vi "Encoder Driver.vi"(11 "UI elements cluster":T1) -> (0 "Error out (no error)":errorcluster)   [LabVIEW 2017]
uses:
  Typedefs/Speed logging states enum.ctl
  Typedefs/UI ctrl refs cluster.ctl
  Typedefs/Laser control knob.ctl
  Typedefs/Frame Size.ctl
  Typedefs/Plane Mode.ctl
  Typedefs/PMT control knob.ctl
  User Interface/Misc/Experiment Type.ctl
  User Interface/Misc/Biology Information.ctl
  Typedefs/HW config states enum.ctl
  Typedefs/Speed window notifier data.ctl
  Typedefs/Notifier Function.ctl
  Typedefs/Speed acq notifier data.ctl
  Global Variables/General Globals.vi
  Global Variables/gl_UI Ctrl Refs.vi
  <vilib>/Utility/tcp.llb/UDP Multicast Read-Write Open.vi
panel:
  out "# elements in queue":i32
  out "PC's IP":string
  out "Loop time (ms)":u32
  out "Loop duration uS":i32
  out "timestamp uS":i32
  out "File path & name":path
  out "State":T2
  out "Closed":bool
  in  "Stop":bool
  in  "Start":bool
  out "Logging interval":u32
  out "Interval of returned values":u32
  in  "Sim":bool
  in  "Stop Button":bool
  out "RPM":dbl(knob) scale=-200.0..200.0
  in  "Path":path=path "C:/Microscope data/April 2014/16 April 2014/Images_16_04_2014"
  out "Chart":dbl(graph)
  out "Angle (Deg)":dbl(knob) scale=0.0..360.0
  # "Simulated Logging Trigger"
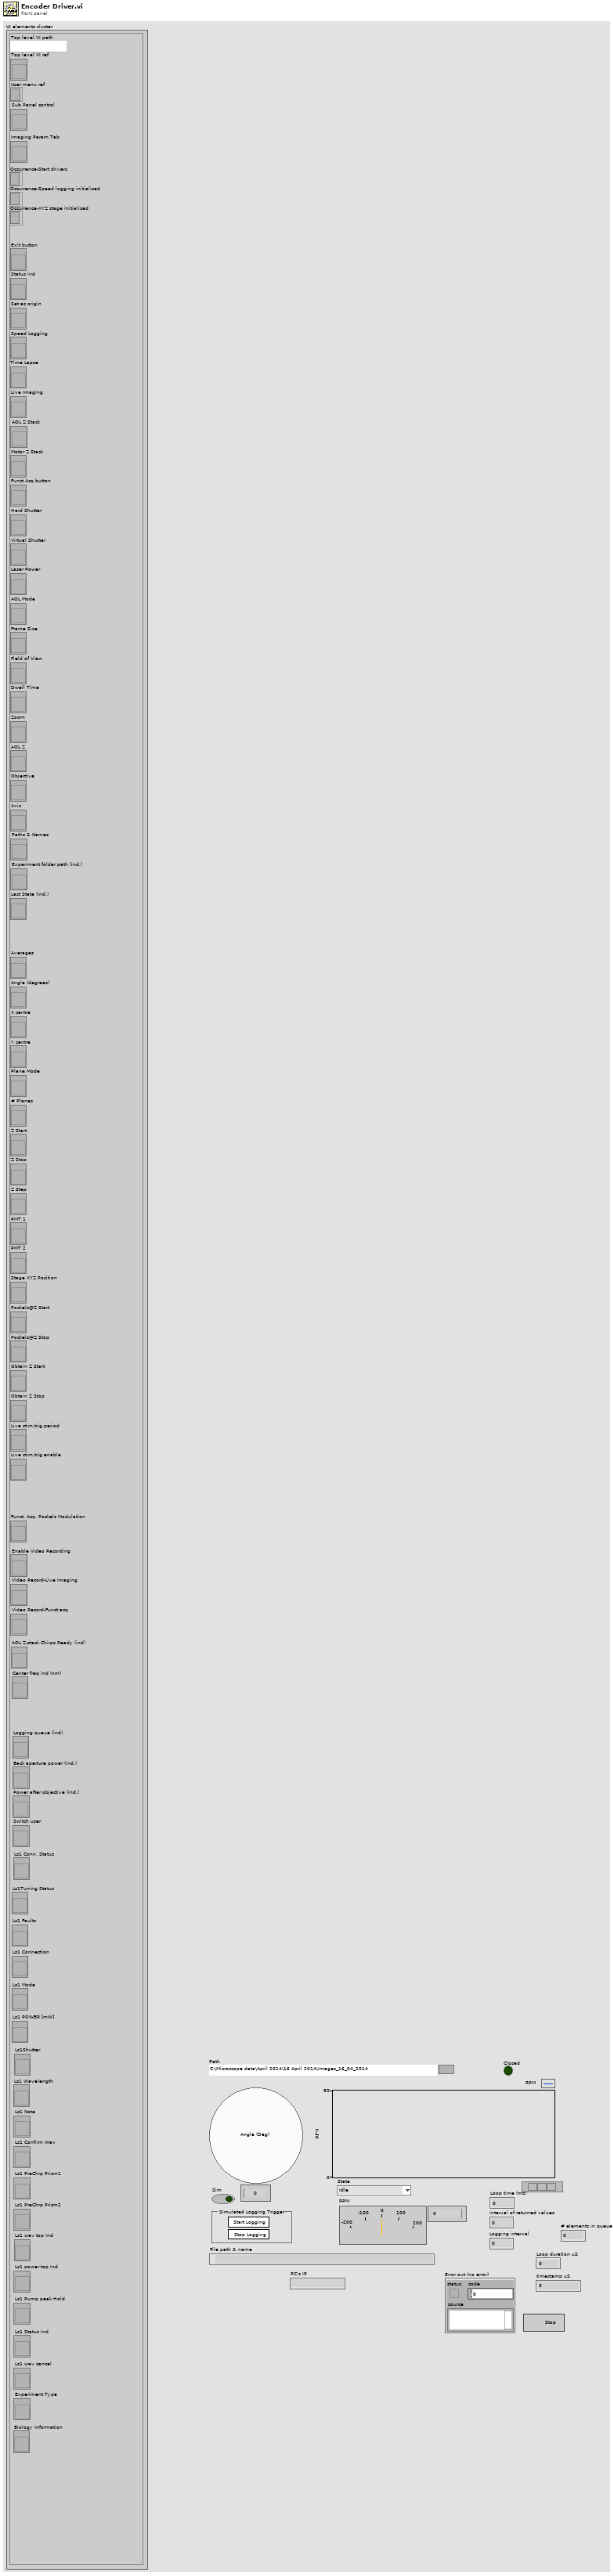
[diagram p1: front panel]
types:
  T1 = typedef "UI ctrl refs cluster.ctl" = cluster{"Top level VI path":path, "Top level VI ref":refnum<vi>, "User menu ref":refnum<k9>, "Sub Panel control":refnum<vi>, "Imaging Param Tab":refnum<vi>, "Occurrence-Start drivers":refnum<k4>, "Occurrence-Speed logging initialised":refnum<k4>, "Occurrence-XYZ stage initialised":refnum<k4>, "Exit button":refnum<vi>, "Status ind":refnum<vi>, "Set as origin":refnum<vi>, "Speed Logging":refnum<vi>, "Time Lapse":refnum<vi>, "Live Imaging":refnum<vi>, "AOL Z Stack":refnum<vi>, "Motor Z Stack":refnum<vi>, "Funct Acq button":refnum<vi>, "Hard Shutter":refnum<vi>, "Virtual Shutter":refnum<vi>, "Laser Power":refnum<vi>, "AOL Mode":refnum<vi>, "Frame Size":refnum<vi>, "Field of View":refnum<vi>, "Dwell Time":refnum<vi>, "Zoom":refnum<vi>, "AOL Z":refnum<vi>, "Objective":refnum<vi>, "Axis":refnum<vi>, "Paths & Names":refnum<vi>, "Experiment folder path (ind.)":refnum<vi>, "Last State (Ind.)":refnum<vi>, "Averages":refnum<vi>, "Angle (degrees)":refnum<vi>, "X centre":refnum<vi>, "Y centre":refnum<vi>, "Plane Mode":refnum<vi>, "# Planes":refnum<vi>, "Z Start":refnum<vi>, "Z Stop":refnum<vi>, "Z Step":refnum<vi>, "PMT 1":refnum<vi>, "PMT 2":refnum<vi>, "Stage XYZ Position":refnum<vi>, "Pockels@Z Start":refnum<vi>, "Pockels@Z Stop":refnum<vi>, "Obtain Z Start":refnum<vi>, "Obtain Z Stop":refnum<vi>, "Live stim.trig.period":refnum<vi>, "Live stim.trig.enable":refnum<vi>, "Funct. Acq. Pockels Modulation":refnum<vi>, "Enable Video Recording":refnum<vi>, "Video Record-Live Imaging":refnum<vi>, "Video Record-Funct acq":refnum<vi>, "AOL Z-stack Chirps Ready (ind)":refnum<vi>, "Center freq ind (nm)":refnum<vi>, "Logging queue (ind)":refnum<vi>, "Back aperture power (ind.)":refnum<vi>, "Power after objective (ind.)":refnum<vi>, "Switch user":refnum<vi>, "Ls1 Conn. Status":refnum<vi>, "Ls1Tuning Status":refnum<vi>, "Ls1 Faults":refnum<vi>, "Ls1 Connection":refnum<vi>, "Ls1 Mode":refnum<vi>, "Ls1 POWER [mW]":refnum<vi>, "Ls1Shutter":refnum<vi>, "Ls1 Wavelength":refnum<vi>, "Ls1 Note":refnum<vi>, "Ls1 Confirm Wav":refnum<vi>, "Ls1 PreChrp Prism1":refnum<vi>, "Ls1 PreChrp Prism2":refnum<vi>, "Ls1 wav top Ind":refnum<vi>, "Ls1 power top Ind":refnum<vi>, "Ls1 Pump peak Hold":refnum<vi>, "Ls1 Status Ind":refnum<vi>, "Ls1 wav cancel":refnum<vi>, "Experiment Type":refnum<vi>, "Biology Information":refnum<vi>}
  T2 = typedef "Speed logging states enum.ctl" = enum16{"Idle", "Open file", "Log", "Close file"}
  T3 = typedef "HW config states enum.ctl" = enum16{"Load from file", "Save to file", "Write all", "Read all", "Write XY stage settings", "Write DAQ FPGA settings", "Write Control FPGA settings", "Write Phys Channels", "Write System Config", "Write HW Config", "Save System Config", "Save HW Config", "Clear", "Compare from file"}
  T4 = typedef "Hardware Configuration settings.ctl" = cluster{"Dev. PC":bool, "Swap XY on stage":bool, "No of AOD":u8, "MC Supported":bool, "Axial MC":bool, "Computer MAC address":string, "Externalise Triggers":bool, "Trigger HW config":T5, "DAQmx Chan":T6, "XY stage available":bool, "XY Stage":T7, "Z stage available":bool, "Z Stage config cluster":T8, "Encoder available":bool, "Encoder":T9, "VidRec available":bool, "Cam VidRec":T10, "Laser Power Control HW config":T11, "Laser 1 available":bool, "Laser 1 config cluster":T12, "Prechirper 1 available":bool, "Prechirper 1 config cluster":T13, "Control system.FPGA available?":bool, "Control Sys. HW config":T14, "DAQ FPGA HW Config":T15}
  T5 = typedef "Triggers HW config.ctl" = cluster{"Available Device List":i32, "Device Address":string}
  T6 = typedef "DAQmx physical channels cluster.ctl" = cluster{"Pockels AO":tag, "Hard shutter AO":tag, "PMT AOs":tag, "Galvo AOs":tag, "Power meter AI":tag}
  T7 = typedef "XY Stage config cluster.ctl" = cluster{"COM port":refnum<visa-resource-name>, "Baudrate":i32, "Type":string}
  T8 = typedef "Z Stage config cluster.ctl" = cluster{"COM port":refnum<visa-resource-name>, "Baudrate":i32, "Type":string}
  T9 = typedef "Encoder config cluster.ctl" = cluster{"IP address":string, "Port":u16, "Wheel radius (cm)":dbl, "Encoder Trigger":tag}
  T10 = typedef "Cam VidRec HW config setup cluster.ctl" = cluster{"DO flag-Video record":tag, "DO flag-Trial start":tag}
  T11 = typedef "Laser Power Control HW config.ctl" = cluster{"Laser Power Control":string, "Laser Power Modulation Control":enum16{"NI", "FPGA"}}
  T12 = typedef "Laser 1 config cluster.ctl" = cluster{"COM port":refnum<visa-resource-name>, "Baud Rate":i32, "Type":string}
  T13 = typedef "PreChirper 1 config cluster.ctl" = cluster{"Type":string, "Baud Rate":i32, "COM port":refnum<visa-resource-name>}
  T14 = typedef "Control Sys HW config cluster.ctl" = cluster{"Control system.FPGA Type":enum16{"Virtex 5", "Virtex 7"}, "Control system.Network adapter name":string, "Control system.MAC address":string, "Control system.Ethernet Port":u32, "Control system.Ethernet Port Opened":bool}
  T15 = typedef "DAQ FPGA HW config cluster.ctl" = cluster{"FGPA Ref":T16, "Target":T17, "input card type":T18}
  T16 = typedef "FPGA Ref.ctl" = refnum<k20>
  T17 = typedef "nirio_resource_hc.ctl" = tag
  T18 = typedef "FPGA input type AC-DC.ctl" = enum16{"AC Card", "DC Card"}
  T19 = typedef "Speed window notifier data.ctl" = cluster{"Angle (Deg)":dbl, "Data value (rpm)":dbl, "Relative time (uS)":i32, "File path":path, "Logging state":T2}
  T20 = typedef "Speed acq notifier data.ctl" = cluster{"Log speed data":bool, "File path":path, "Initial timestamp":timestamp}
  T21 = typedef "Notifier Function.ctl" = enum16{"Send notifier", "Wait on notification", "Release notifier"}
  T22 = enum16{"open", "replace", "create", "open or create", "replace or create", "replace or create with confirmation"}
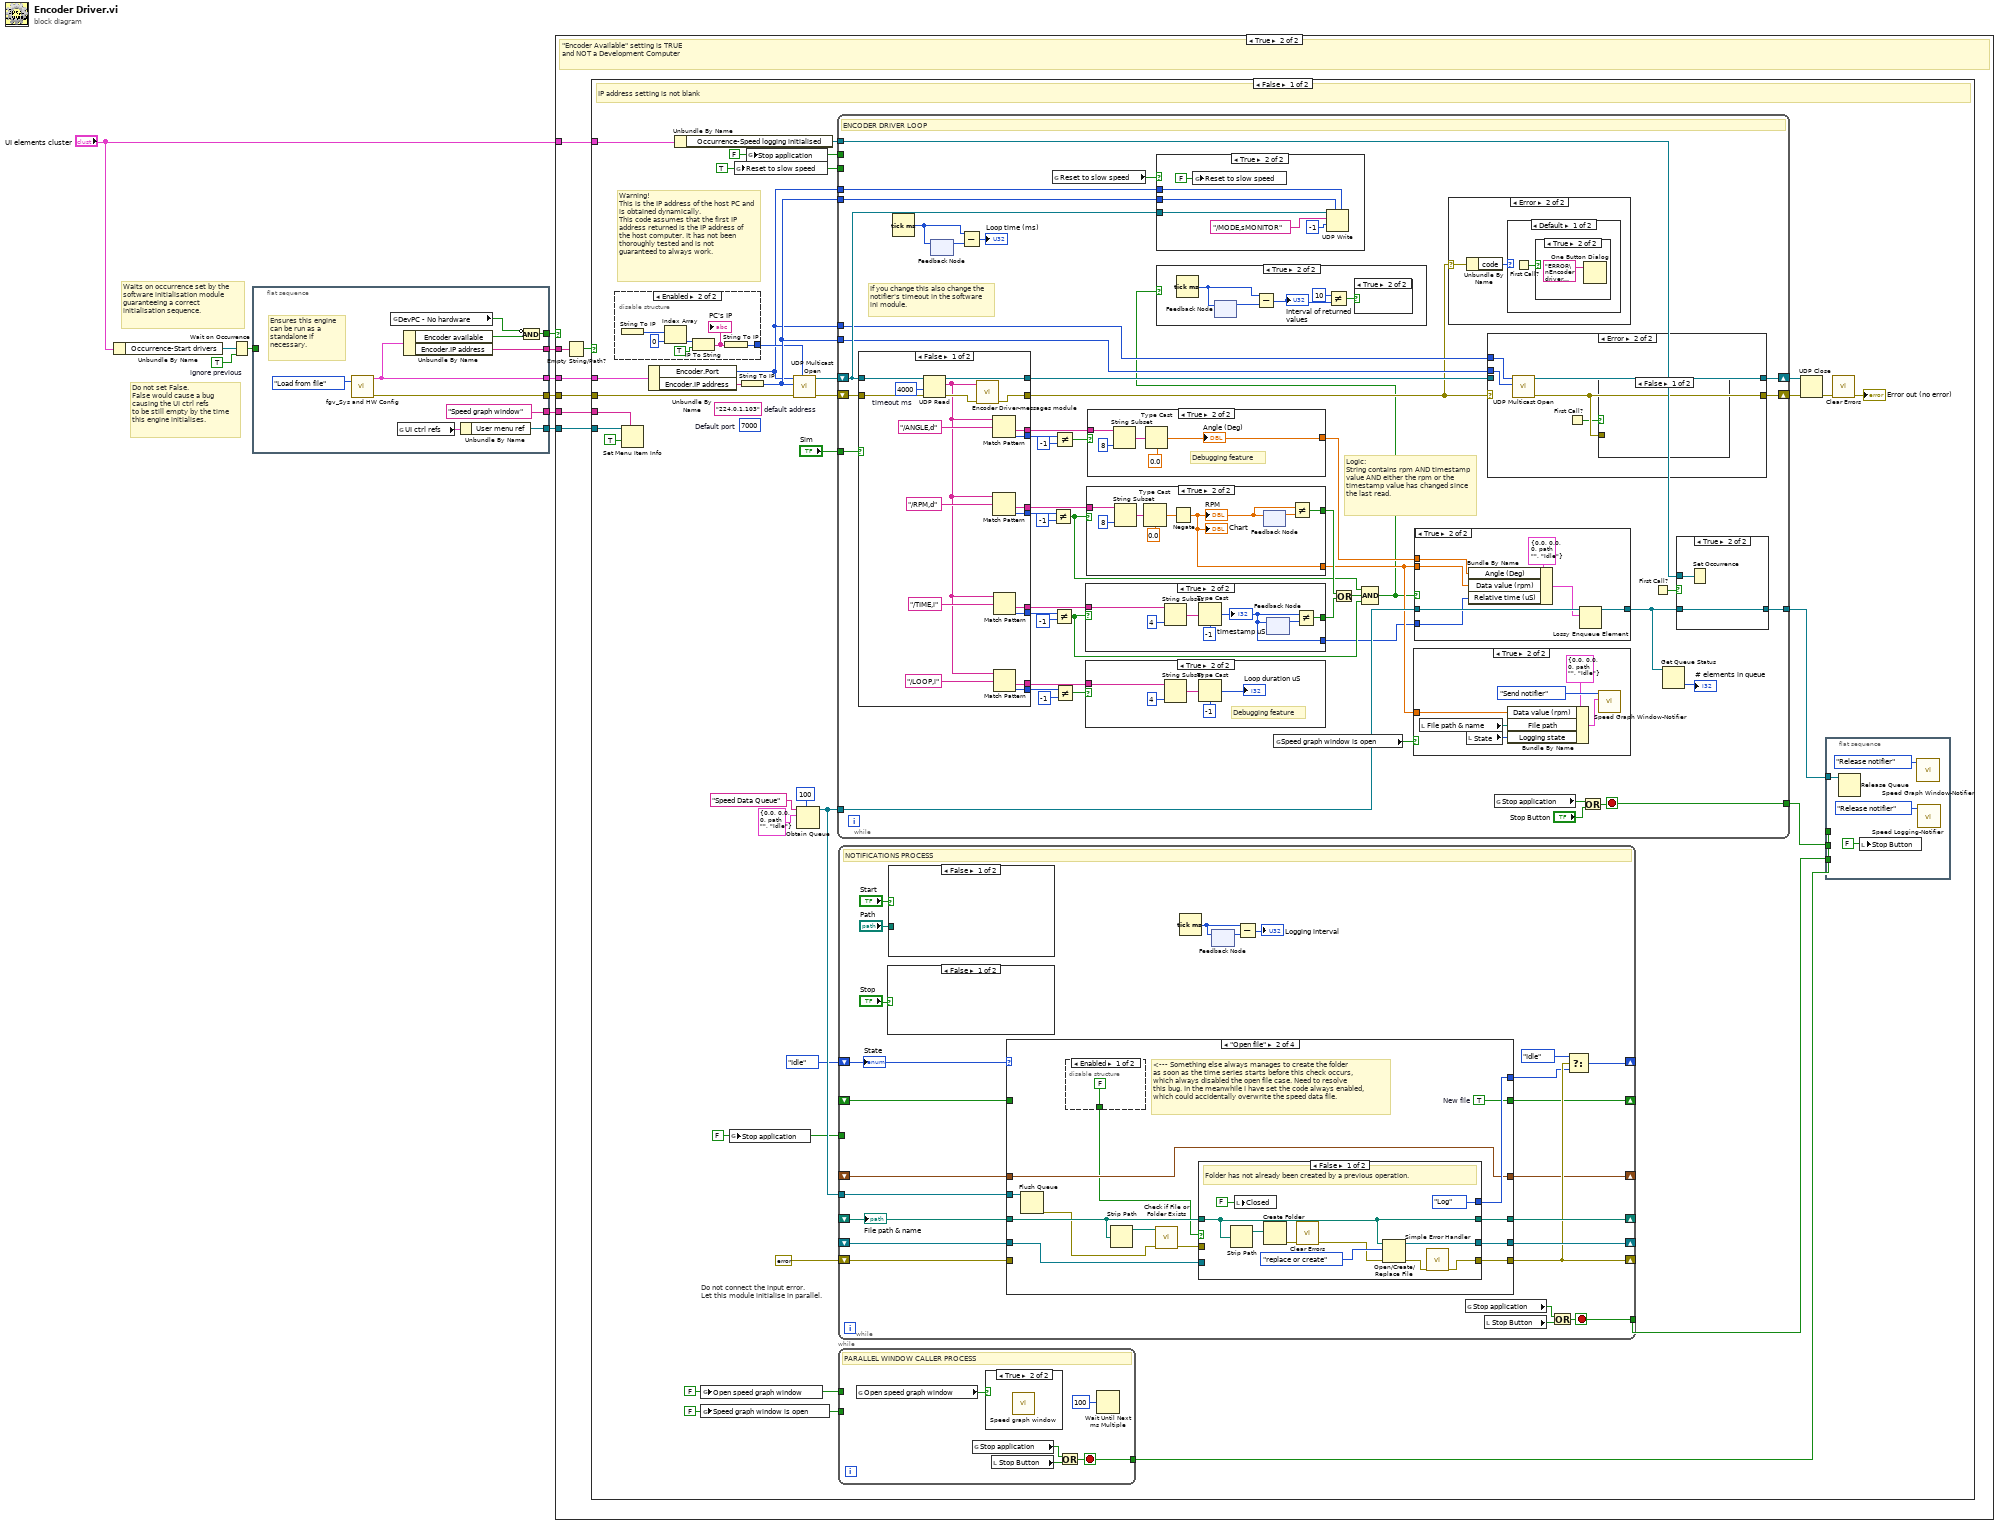
[diagram p0: block diagram]
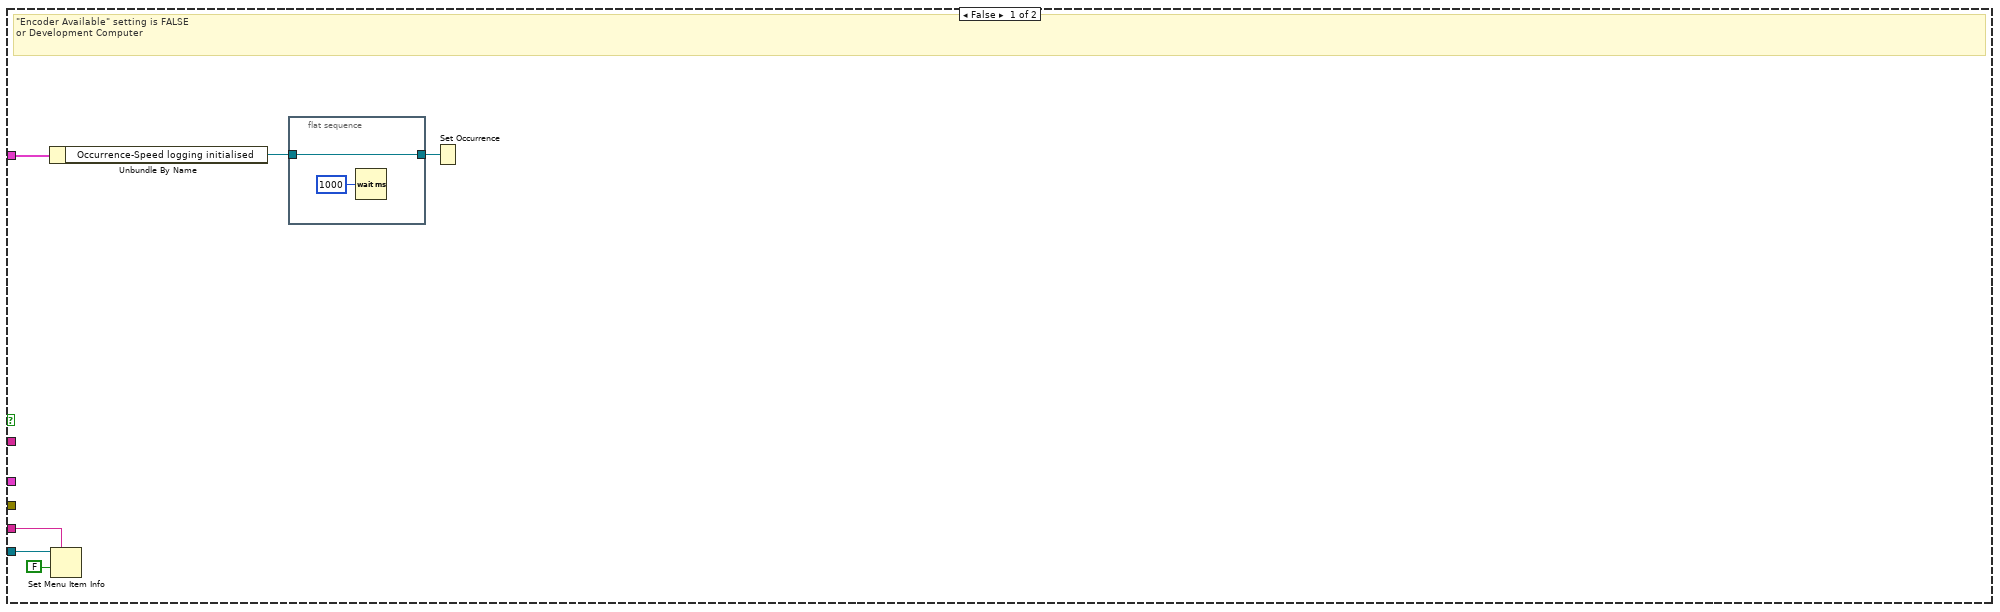
[diagram p2: hidden frame]
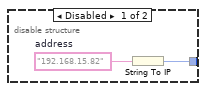
[diagram p3: hidden frame]
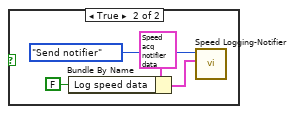
[diagram p5: hidden frame]
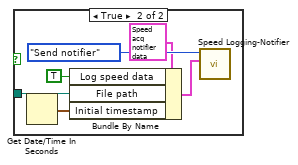
[diagram p6: hidden frame]
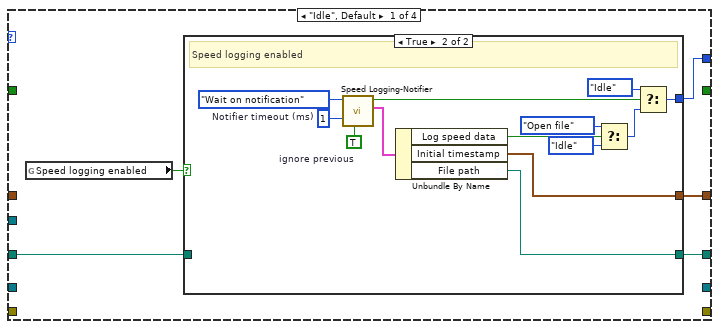
[diagram p7: hidden frame]
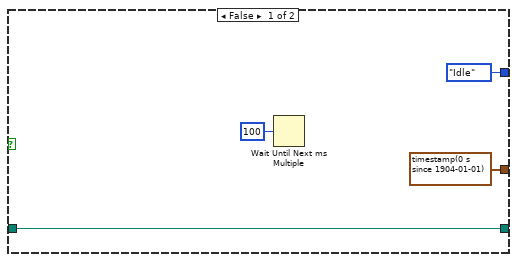
[diagram p8: hidden frame]
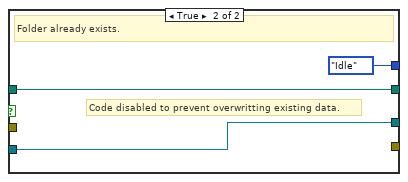
[diagram p10: hidden frame]
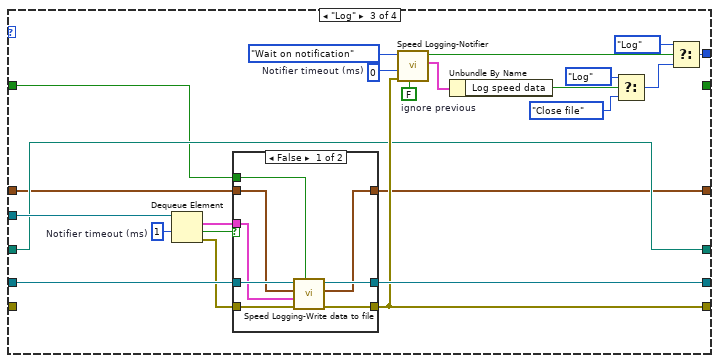
[diagram p11: hidden frame]
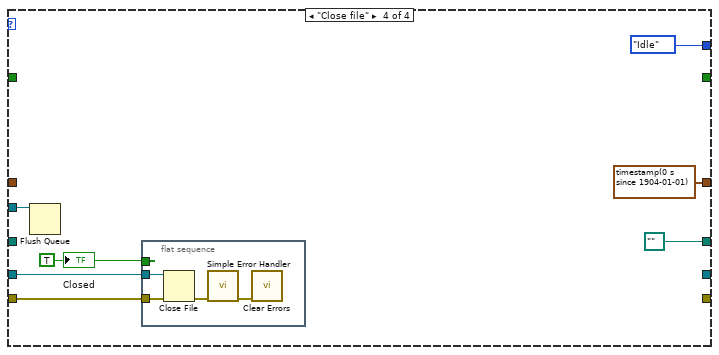
[diagram p13: hidden frame]
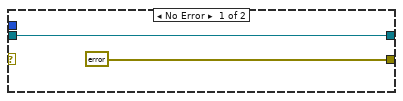
[diagram p14: hidden frame]
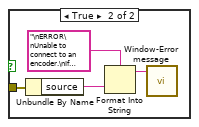
[diagram p15: hidden frame]
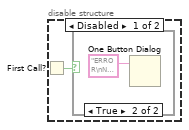
[diagram p20: hidden frame]
diagram:
  w6 = TRUE  # ignore previous
  # "Do not set False.\nFalse would cause a bug\ncausing the UI ctrl refs\nto be still empty by the time\nthis engine initialises."
  # "Waits on occurrence set by the software initialisation module guaranteeing a correct initialisation sequence."
  n1 = Unbundle By Name("UI elements cluster") -> ("Occurrence-Start drivers"=w4:refnum<k4>)
  n2 = Wait on Occurrence(1:w6, 2:w4) -> (0:w5:bool)  [unwired: 1 in]
  n3 = flat-sequence {
    tunnel: [w19] -> w10
    tunnel: [w18] -> w9
    tunnel: [w17] -> w8
    tunnel: [w14] -> w7
    tunnel: w5 -> [_]
    tunnel: [w12] -> w2
    tunnel: ["Speed graph window"] -> w1
    frame #0 {
      # "Ensures this engine can be run as a standalone if necessary."
      n4 = call "fgv_Sys and HW Config.vi"("Function"=HW_config_states_enum."Load from file") -> ("error out"=w19:errorcluster, "Hardware Configuration OUT"=w18:T4)  [unwired: 8 in, 1 out]
      n5 = global read "General Globals.vi" "DevPC - No hardware"() -> (w15:bool)
      n6 = global read "gl_UI Ctrl Refs.vi" "UI ctrl refs"() -> (w13:T1)
      n7 = Unbundle By Name(w18) -> ("Encoder available"=w16:bool, "Encoder.IP address"=w17:string)
      n8 = Unbundle By Name(w13) -> ("User menu ref"=w12:refnum<k9>)
      n9 = Compound Arithmetic op=AND(invert w15, w16) -> (w14:bool)
    }
  }
  n10 = case shown="True" w7 {
    tunnel: "UI elements cluster" -> [w26 w35]
    tunnel: w10 -> [_ w34]
    tunnel: w9 -> [_ w33]
    tunnel: w8 -> [_ w32]
    tunnel: w2 -> [w21 w30]
    tunnel: w1 -> [w22 w29]
    frame False {
      # "\"Encoder Available\" setting is FALSE\nor Development Computer"
      n11 = Unbundle By Name(w26) -> ("Occurrence-Speed logging initialised"=w25:refnum<k4>)
      n12 = Set Menu Item Info(7:w22, 9:FALSE ("enabled"), 11:w21) -> ()  [unwired: 2 in, 4 out]
      n13 = flat-sequence {
        tunnel: w25 -> [w27]
        tunnel: [w27] -> w24
        frame #0 {
          n14 = Wait (ms)(milliseconds to wait=u32 1000) -> ()  [unwired: 1 out]
        }
      }
      n15 = Set Occurrence(w24) -> ()
    }
    frame True {
      # "\"Encoder Available\" setting is TRUE\nand NOT a Development Computer"
      n16 = Empty String/Path?(string/path=w32) -> (empty?=w31:bool)
      n17 = case shown="False" w31 {
        tunnel: w35 -> [w47 _]
        tunnel: w34 -> [w43 _]
        tunnel: w33 -> [w41 _]
        tunnel: w30 -> [w37 w368]
        tunnel: w29 -> [w38 w366]
        frame False {
          w46 = FALSE ("Stop application")
          w58 = TRUE ("Reset to slow speed")
          w53 = FALSE ("Stop application")
          (unwired) u16 7000  # Default port
          (unwired) "224.0.1.103"  # default address
          w51 = FALSE ("Speed graph window is open")
          w52 = FALSE ("Open speed graph window")
          # "Do not connect the input error.\nLet this module initialise in parallel."
          # "Warning!\nThis is the IP address of the host PC and is obtained dynamically.\nThis code assumes that the first IP address returned is the IP address of the host computer. It has not been thoroughly tested and is not guaranteed to always work."
          # "IP address setting is not blank"
          n18 = disable-structure shown="Enabled" {
            disable-tunnel: [w69 w71] -> w50
            frame Disabled {
              w70 = "192.168.15.82"  # address
              n19 = String To IP(1:w70) -> (0:w69:u32)
            }
            frame Enabled {
              n20 = String To IP() -> (0:w72:u32[])  [unwired: 1 in]
              n21 = Index Array(array=w72, index=0) -> (element=w74:u32)
              n22 = IP To String(1:TRUE ("dot notation? (F)"), 2:w74) -> (0:w76:string)
              "PC's IP" <- w76
              n23 = String To IP(1:w76) -> (0:w71:u32)
            }
          }
          n24 = Set Menu Item Info(7:w38, 9:TRUE ("enabled"), 11:w37) -> ()  [unwired: 2 in, 4 out]
          n25 = Unbundle By Name(w41) -> ("Encoder.Port"=w44:u16, "Encoder.IP address"=w45:string)
          n26 = Unbundle By Name(w47) -> ("Occurrence-Speed logging initialised"=w49:refnum<k4>)
          n27 = global write "General Globals.vi" "Open speed graph window"(w52) -> ()
          n28 = global write "General Globals.vi" "Speed graph window is open"(w51) -> ()
          n29 = global write "General Globals.vi" "Stop application"(w53) -> ()
          n30 = global write "General Globals.vi" "Reset to slow speed"(w58) -> ()
          n31 = String To IP(1:w45) -> (0:w57:u32)
          n32 = global write "General Globals.vi" "Stop application"(w46) -> ()
          n33 = call-poly <vilib>:"UDP Multicast Open.vi"("net address"=w50, "error in (no error)"=w43, "multicast addr"=w57, "port"=w44) -> ("error out"=w59:errorcluster, "connection ID"=w62:refnum<k16>)  [unwired: 5 in, 1 out]
          n34 = Obtain Queue(max queue size (-1, unlimited)=100, name (unnamed)="Speed Data Queue", element data type=T19 {"Angle (Deg)"=0.0, "Data value (rpm)"=0.0, "Relative time (uS)"=0, "File path"=path "", "Logging state"=enum."Idle"} ("Speed window data")) -> (queue out=w66:refnum<queue>)  [unwired: 2 in, 2 out]
          n35 = while {
            tunnel: "Sim" -> [w257]
            tunnel: [w252] -> w68
            tunnel: w66 -> [w253]
            tunnel: [w227] -> w65
            tunnel: w57 -> [w250]
            tunnel: w44 -> [w249]
            tunnel: w58 -> [_]
            tunnel: w49 -> [w225]
            tunnel: w57 -> [w223]
            tunnel: w44 -> [w222]
            shift-right: [w221] -> w56
            shift-left: w62 -> [w248]
            shift-right: [w220] -> w55
            shift-left: w59 -> [w228]
            tunnel: w46 -> [_]
            stop <- w252 stop-if-true
            # "If you change this also change the notifier's timeout in the software ini module."
            # "Logic:\nString contains rpm AND timestamp value AND either the rpm or the timestamp value has changed since the last read."
            # "ENCODER DRIVER LOOP"
            n36 = case shown="False" w257 {
              tunnel: w248 -> [w352 w365]
              tunnel: [w350 w362] -> w261
              tunnel: [w348 w365] -> w219
              tunnel: [w347 w360] -> w260
              tunnel: [w345 w360] -> w259
              tunnel: [w344 w362] -> w258
              tunnel: w228 -> [w343 w364]
              tunnel: [w335 w364] -> w218
              tunnel: [w340 w360] -> w246
              tunnel: [w339 w360] -> w244
              tunnel: [w338 w361] -> w243
              tunnel: [w337 w362] -> w242
              frame False {
                w346 = 4000  # timeout ms
                n37 = UDP Read(connection ID=w352, timeout ms (25000)=w346, 8:w343) -> (data out=w334:string, error out=w336:errorcluster, 3:w348:refnum<k16>)  [unwired: 1 in, 2 out]
                n38 = call "Encoder Driver-messages module.vi"("error in (no error)"=w336, "Command/Response string"=w334) -> ("error"=w335:errorcluster)  [unwired: 9 in]
                n39 = Match Pattern(string=w334, regular expression="/ANGLE,d" ("format string")) -> (after substring=w350:string, offset past match=w347:i32)  [unwired: 1 in, 2 out]
                n40 = Match Pattern(string=w334, regular expression="/RPM,d" ("format string")) -> (after substring=w344:string, offset past match=w345:i32)  [unwired: 1 in, 2 out]
                n41 = Match Pattern(string=w334, regular expression="/TIME,i" ("format string")) -> (after substring=w338:string, offset past match=w340:i32)  [unwired: 1 in, 2 out]
                n42 = Match Pattern(string=w334, regular expression="/LOOP,i" ("format string")) -> (after substring=w337:string, offset past match=w339:i32)  [unwired: 1 in, 2 out]
              }
              frame True {
                w360 = 0 ("offset past match")
                n43 = feedback #1() -> (w358:i32)  [unwired: 1 in]
                n44 = Increment(x=w358) -> (x+1=w359:i32)
                n45 = To Long Integer(number=w359) -> (32bit integer=w353:i32)
                n46 = feedback-in #1(w353) -> ()
                n47 = Equal?(x=2147483647 ("32bit integer"), y=w353) -> (x = y?=w356:bool)
                n48 = Random Number (0-1)() -> (number: 0 to 1=w363:dbl)
                n49 = Select(t=0 ("32bit integer"), s=w356, f=w353) -> (s? t:f=w354:i32)
                n50 = Format Into String(w363) -> (resulting string=w362:string)  [unwired: 3 in, 1 out]
                n51 = Format Into String(w354) -> (resulting string=w361:string)  [unwired: 3 in, 1 out]
              }
            }
            n52 = Tick Count (ms)() -> (millisecond timer value=w231:u32)
            n53 = feedback #2() -> (w230:u32)  [unwired: 1 in]
            n54 = feedback-in #2(w231) -> ()
            n55 = Subtract(x=w231, y=w230) -> (x-y=→"Loop time (ms)":u32)
            n56 = Not Equal?(x=w259, y=-1) -> (x != y?=w237:bool)
            n57 = global read "General Globals.vi" "Reset to slow speed"() -> (w232:bool)
            n58 = Not Equal?(x=w246, y=-1) -> (x != y?=w239:bool)
            n59 = Not Equal?(x=w260, y=-1) -> (x != y?=w255:bool)
            n60 = Not Equal?(x=w244, y=-1) -> (x != y?=w241:bool)
            n61 = case shown="True" w239 {
              tunnel: w243 -> [_ w291]
              tunnel: [FALSE w289] -> w240
              tunnel: [_ w288] -> w234
              frame False {
              }
              frame True {
                n62 = String Subset(string=w291, length (rest)=4 ("length (rest)")) -> (substring=w292:string)  [unwired: 1 in]
                n63 = Type Cast(type=-1 ("y"), x=w292) -> (*(type *) &x=w288:i32)
                "timestamp uS" <- w288
                n64 = feedback #3() -> (w290:i32)  [unwired: 1 in]
                n65 = feedback-in #3(w288) -> ()
                n66 = Not Equal?(x=w288, y=w290) -> (x != y?=w289:bool)
              }
            }
            n67 = case shown="True" w241 {
              tunnel: w242 -> [_ w283]
              frame False {
              }
              frame True {
                # "Debugging feature"
                n68 = String Subset(string=w283, length (rest)=4 ("length (rest)")) -> (substring=w284:string)  [unwired: 1 in]
                n69 = Type Cast(type=-1 ("y"), x=w284) -> (*(type *) &x=→"Loop duration uS":i32)
              }
            }
            n70 = case shown="True" w237 {
              tunnel: w258 -> [_ w303]
              tunnel: [FALSE w302] -> w238
              tunnel: [_ w296] -> w235
              frame False {
              }
              frame True {
                n71 = String Subset(string=w303, length (rest)=8 ("length (rest)")) -> (substring=w298:string)  [unwired: 1 in]
                n72 = Type Cast(type=0.0 ("number"), x=w298) -> (*(type *) &x=w297:dbl)
                n73 = Negate(x=w297) -> (-x=w296:dbl)
                "Chart" <- w296
                "RPM" <- w296
                n74 = feedback #4() -> (w300:dbl)  [unwired: 1 in]
                n75 = feedback-in #4(w296) -> ()
                n76 = Not Equal?(x=w296, y=w300) -> (x != y?=w302:bool)
              }
            }
            n77 = case shown="True" w255 {
              tunnel: w261 -> [_ w331]
              tunnel: [_ w329] -> w233
              frame False {
              }
              frame True {
                # "Debugging feature"
                n78 = String Subset(string=w331, length (rest)=8 ("length (rest)")) -> (substring=w330:string)  [unwired: 1 in]
                n79 = Type Cast(type=0.0 ("number"), x=w330) -> (*(type *) &x=w329:dbl)
                "Angle (Deg)" <- w329
              }
            }
            n80 = case shown="True" w232 {
              tunnel: w248 -> [_ w313]
              tunnel: w249 -> [_ w312]
              tunnel: w250 -> [_ w311]
              frame False {
              }
              frame True {
                n81 = global write "General Globals.vi" "Reset to slow speed"(FALSE ("Reset to slow speed")) -> ()
                n82 = UDP Write(address=w311, port or service name=w312, connection ID=w313, data in="/MODE,sMONITOR", 9:-1 ("timeout ms (25000)")) -> ()  [unwired: 1 in, 2 out]
              }
            }
            n83 = global read "General Globals.vi" "Speed graph window is open"() -> (w214:bool)
            n84 = Or(x=w238, y=w240) -> (x .or. y?=w236:bool)
            n85 = Compound Arithmetic op=AND(w237, w236, w239) -> (w215:bool)
            n86 = case shown="True" w215 {
              frame False {
              }
              frame True {
                n87 = Tick Count (ms)() -> (millisecond timer value=w327:u32)
                n88 = feedback #5() -> (w328:u32)  [unwired: 1 in]
                n89 = feedback-in #5(w327) -> ()
                n90 = Subtract(x=w327, y=w328) -> (x-y=w326:u32)
                "Interval of returned values" <- w326
                n91 = Not Equal?(x=u32 10, y=w326) -> (x != y?=w324:bool)
                n92 = case shown="True" w324 {
                  frame False {
                  }
                  frame True {
                  }
                }
              }
            }
            n93 = case shown="True" w214 {
              tunnel: w235 -> [_ w305]
              frame False {
              }
              frame True {
                n94 = local read "File path & name"() -> (w307:path)
                n95 = local read "State"() -> (w304:T2)
                n96 = Bundle By Name(cluster=T19 {"Angle (Deg)"=0.0, "Data value (rpm)"=0.0, "Relative time (uS)"=0, "File path"=path "", "Logging state"=enum."Idle"} ("Speed window data"), "Data value (rpm)"=w305, "File path"=w307, "Logging state"=w304) -> (w306:T19)
                n97 = call "Speed Graph Window-Notifier.vi"("Speed window data"=w306, "Notifier Function"=Notifier_Function."Send notifier") -> ()  [unwired: 7 in, 3 out]
              }
            }
            n98 = case shown="True" w215 {
              tunnel: w253 -> [w316 w323]
              tunnel: [w316 w322] -> w217
              tunnel: w235 -> [_ w319]
              tunnel: w234 -> [_ w318]
              tunnel: w233 -> [_ w317]
              frame False {
              }
              frame True {
                n99 = Bundle By Name(cluster=T19 {"Angle (Deg)"=0.0, "Data value (rpm)"=0.0, "Relative time (uS)"=0, "File path"=path "", "Logging state"=enum."Idle"} ("Speed window data"), "Angle (Deg)"=w317, "Data value (rpm)"=w319, "Relative time (uS)"=w318) -> (w320:T19)
                n100 = Lossy Enqueue Element(queue=w323, element=w320) -> (queue out=w322:refnum<queue>)  [unwired: 1 in, 3 out]
              }
            }
            n101 = case shown="Error" w218 {
              selector: w218 -> [_ w277]
              frame No Error {
              }
              frame Error {
                n102 = Unbundle By Name(w277) -> ("code"=w276:i32)
                n103 = case shown="Default" w276 {
                  frame Default {
                    n104 = First Call?() -> (First Call?: T/F=w278:bool)
                    n105 = case shown="True" w278 {
                      frame False {
                      }
                      frame True {
                        n106 = One Button Dialog(message="ERROR\nEncoder driver comms error.") -> ()  [unwired: 1 in, 1 out]
                      }
                    }
                  }
                  frame 56 {
                    n107 = disable-structure shown="Enabled" {
                      frame Disabled {
                        n108 = First Call?() -> (First Call?: T/F=w280:bool)
                        n109 = case shown="True" w280 {
                          frame False {
                          }
                          frame True {
                            n110 = One Button Dialog(message="ERROR\nNo encoder present.") -> ()  [unwired: 1 in, 1 out]
                          }
                        }
                      }
                      frame Enabled {
                      }
                    }
                  }
                }
              }
            }
            n111 = case shown="Error" w218 {
              tunnel: w223 -> [_ w268]
              tunnel: w222 -> [_ w267]
              tunnel: [w263 w266] -> w221
              tunnel: [errorcluster {"status"=FALSE, "code"=0, "source"=""} ("error out") w265] -> w220
              tunnel: w219 -> [w263 _]
              frame No Error {
              }
              frame Error {
                n112 = call-poly <vilib>:"UDP Multicast Open.vi"("multicast addr"=w268, "port"=w267) -> ("error out"=w265:errorcluster, "connection ID"=w266:refnum<k16>)  [unwired: 7 in, 1 out]
                n113 = First Call?() -> (First Call?: T/F=w264:bool)
                n114 = case shown="False" w264 {
                  tunnel: w265 -> [_ w272]
                  frame False {
                  }
                  frame True {
                    n115 = Unbundle By Name(w272) -> ("source"=w271:string)
                    n116 = Format Into String(format string="\nERROR\nUnable to connect to an encoder.\nIf there is an encoder physically connected to the system carry out the following steps to rectify the issue:\n1. Shut down the software.\n2. Power down the AOL control unit and the encoder driver unit by disconnecting its USB power supply cable.\n3. Power up the encoder driver unit and wait until its LED becomes green.\n4. Start the software.\n5. Power up the AOL control unit and wait for 10 seconds before you use the software for imaging.\n\nERROR SOURCE:\n%s\n\nCheck the firewall!", w271) -> (resulting string=w270:string)  [unwired: 2 in, 1 out]
                    n117 = call "Window-Error message.vi"("Message"=w270) -> ()  [unwired: 10 in, 1 out]
                  }
                }
              }
            }
            n118 = global read "General Globals.vi" "Stop application"() -> (w224:bool)
            n119 = Or(x=w224, y="Stop Button") -> (x .or. y?=w252:bool)
            n120 = First Call?() -> (First Call?: T/F=w226:bool)
            n121 = Get Queue Status(queue=w217) -> (# elements in queue=→"# elements in queue":i32)  [unwired: 2 in, 7 out]
            n122 = case shown="True" w226 {
              tunnel: w217 -> [w273 w275]
              tunnel: [w273 w275] -> w227
              tunnel: w225 -> [_ w274]
              frame False {
              }
              frame True {
                n123 = Set Occurrence(w274) -> ()
              }
            }
          }
          n124 = while {
            tunnel: w52 -> [_]
            tunnel: w51 -> [_]
            tunnel: [w77] -> w40
            stop <- w77 stop-if-true
            # "PARALLEL WINDOW CALLER PROCESS"
            n125 = global read "General Globals.vi" "Open speed graph window"() -> (w78:bool)
            n126 = global read "General Globals.vi" "Stop application"() -> (w80:bool)
            n127 = case shown="True" w78 {
              frame False {
              }
              frame True {
                n128 = call "Speed graph window.vi"() -> ()  [unwired: 12 in]
              }
            }
            n129 = local read "Stop Button"() -> (w81:bool)
            n130 = Or(x=w80, y=w81) -> (x .or. y?=w77:bool)
            n131 = Wait Until Next ms Multiple(millisecond multiple=u32 100 ("millisecond timer value")) -> ()  [unwired: 1 out]
          }
          n132 = while {
            shift-right: [w104] -> _
            shift-left: _ -> [w103]
            shift-right: [w99] -> _
            shift-left: errorcluster {"status"=FALSE, "code"=0, "source"=""} ("error in (no error)") -> [w102]
            shift-right: [w98] -> _
            shift-left: Speed_logging_states_enum."Idle" ("States") -> [w105]
            shift-right: [w101] -> _
            shift-left: _ -> [w100]
            tunnel: [w88] -> w67
            tunnel: w66 -> [w91]
            shift-right: [w84] -> _
            shift-left: _ -> [w85]
            shift-right: [w83] -> _
            shift-left: _ -> [w82]
            tunnel: w53 -> [_]
            stop <- w88 stop-if-true
            # "NOTIFICATIONS PROCESS"
            n133 = case shown="False" "Stop" {
              frame False {
              }
              frame True {
                n134 = Bundle By Name(cluster=T20 {"Log speed data"=TRUE, "File path"=path "", "Initial timestamp"=timestamp(0 s since 1904-01-01)} ("Value to send"), "Log speed data"=FALSE ("Log?")) -> (w106:T20)
                n135 = call "Speed Logging-Notifier.vi"("Value to send"=w106, "Notifier Function"=Notifier_Function."Send notifier") -> ()  [unwired: 7 in, 3 out]
              }
            }
            n136 = case shown="False" "Start" {
              tunnel: "Path" -> [_ w112]
              frame False {
              }
              frame True {
                n137 = Get Date/Time In Seconds() -> (seconds since 1Jan1904=w110:timestamp)
                n138 = Bundle By Name(cluster=T20 {"Log speed data"=TRUE, "File path"=path "", "Initial timestamp"=timestamp(0 s since 1904-01-01)} ("Value to send"), "Log speed data"=TRUE ("Log?"), "File path"=w112, "Initial timestamp"=w110) -> (w111:T20)
                n139 = call "Speed Logging-Notifier.vi"("Value to send"=w111, "Notifier Function"=Notifier_Function."Send notifier") -> ()  [unwired: 7 in, 3 out]
              }
            }
            n140 = case shown="\"Open file\"" w105 {
              tunnel: [_ w150 w187 _] -> w104
              tunnel: w103 -> [_ w138 w186 w204]
              tunnel: [_ w149 w178 _] -> w99
              tunnel: w102 -> [_ _ _ w203]
              tunnel: [w120 w147 w179 Speed_logging_states_enum."Idle" ("States")] -> w97
              tunnel: [w119 w148 w169 path "" ("appended path")] -> w101
              tunnel: w100 -> [w118 w145 w169 _]
              tunnel: w91 -> [_ w140 w177 w199]
              tunnel: w85 -> [_ w143 w166 _]
              tunnel: [w116 w143 w165 timestamp(0 s since 1904-01-01) ("seconds since 1Jan1904")] -> w84
              tunnel: [_ w142 _ _] -> w83
              tunnel: w82 -> [_ _ w167 _]
              frame "Idle", Default {
                n141 = global read "General Globals.vi" "Speed logging enabled"() -> (w117:bool)
                n142 = case shown="True" w117 {
                  tunnel: [Speed_logging_states_enum."Idle" ("f") w137] -> w120
                  tunnel: [w123 w125] -> w119
                  tunnel: w118 -> [w123 _]
                  tunnel: [timestamp(0 s since 1904-01-01) ("seconds since 1Jan1904") w126] -> w116
                  frame False {
                    n143 = Wait Until Next ms Multiple(millisecond multiple=u32 100) -> ()  [unwired: 1 out]
                  }
                  frame True {
                    w127 = 1  # Notifier timeout (ms)
                    w130 = TRUE  # ignore previous
                    # "Speed logging enabled"
                    n144 = call "Speed Logging-Notifier.vi"("ignore previous (F)"=w130, "Timeout waiting in ms (-1)"=w127, "Notifier Function"=Notifier_Function."Wait on notification") -> ("Notification data received"=w129:T20, "Timed out waiting"=w131:bool)  [unwired: 6 in, 1 out]
                    n145 = Unbundle By Name(w129) -> ("Log speed data"=w128:bool, "Initial timestamp"=w126:timestamp, "File path"=w125:path)
                    n146 = Select(t=Speed_logging_states_enum."Open file" ("f"), s=w128, f=Speed_logging_states_enum."Idle") -> (s? t:f=w133:T2)
                    n147 = Select(t=Speed_logging_states_enum."Idle" ("States"), s=w131, f=w133) -> (s? t:f=w137:T2)
                  }
                }
              }
              frame "Open file" {
                w142 = TRUE  # New file
                # "<--- Something else always manages to create the folder\nas soon as the time series starts before this check occurs,\nwhich always disabled the open file case. Need to resolve\nthis bug. In the meanwhile I have set the code always enabled,\nwhich could accidentally overwrite the speed data file."
                n148 = Flush Queue(queue=w140) -> (error out=w139:errorcluster)  [unwired: 1 in, 2 out]
                n149 = disable-structure shown="Enabled" {
                  disable-tunnel: [FALSE _] -> w141
                  frame Enabled {
                  }
                  frame Disabled {
                  }
                }
                n150 = Strip Path(path=w145) -> (stripped path=w144:path)  [unwired: 1 out]
                n151 = call <vilib>:"Check if File or Folder Exists.vi"("error in (no error)"=w139, "path"=w144) -> ("error out"=w146:errorcluster)  [unwired: 7 in, 2 out]
                n152 = case shown="False" w141 {
                  tunnel: [w160 w162] -> w150
                  tunnel: [w158 _] -> w149
                  tunnel: [w153 w164] -> w148
                  tunnel: w145 -> [w153 w164]
                  tunnel: [Speed_logging_states_enum."Log" ("States") Speed_logging_states_enum."Idle" ("States")] -> w147
                  tunnel: w146 -> [_ _]
                  tunnel: w138 -> [_ w162]
                  frame False {
                    # "Folder has not already been created by a previous operation."
                    n153 = Strip Path(path=w153) -> (stripped path=w154:path)  [unwired: 1 out]
                    n154 = local write "Closed"(FALSE ("Closed")) -> ()
                    n155 = Create Folder(path (use dialog)=w154) -> (error out=w157:errorcluster)  [unwired: 2 in, 2 out]
                    n156 = call <vilib>:"Clear Errors.vi"("error in (no error)"=w157) -> ("error out"=w152:errorcluster)  [unwired: 5 in, 1 out]
                    n157 = Open/Create/Replace File(file path (use dialog)=w153, error in=w152, operation (0:open)=T22."replace or create") -> (refnum out=w160:refnum<file>, error out=w159:errorcluster)  [unwired: 3 in, 1 out]
                    n158 = call <vilib>:"Simple Error Handler.vi"("error in (no error)"=w159) -> ("error out"=w158:errorcluster)  [unwired: 4 in, 4 out]
                  }
                  frame True {
                    # "Code disabled to prevent overwritting existing data."
                    # "Folder already exists."
                  }
                }
              }
              frame "Log" {
                w172 = 0  # Notifier timeout (ms)
                w173 = 1  # Notifier timeout (ms)
                w176 = FALSE  # ignore previous
                n159 = Dequeue Element(queue=w177, timeout in ms (-1)=w173) -> (element=w168:T19, timed out?=w171:bool, error out=w170:errorcluster)  [unwired: 1 in, 1 out]
                n160 = case shown="False" w171 {
                  tunnel: [w195 w197] -> w187
                  tunnel: w186 -> [w194 w197]
                  tunnel: [w193 w198] -> w178
                  tunnel: w170 -> [w192 w198]
                  tunnel: w168 -> [w191 _]
                  tunnel: w166 -> [w190 w196]
                  tunnel: w167 -> [w189 _]
                  tunnel: [w188 w196] -> w165
                  frame False {
                    n161 = call "Speed Logging-Write data to file.vi"("New file"=w189, "error in (no error)"=w192, "Speed window data"=w191, "Timestamp at trial start"=w190, "Byte Stream File in"=w194) -> ("error out"=w193:errorcluster, "Timestamp at trial start"=w188:timestamp, "Byte Stream File out"=w195:refnum<file>)  [unwired: 4 in]
                  }
                  frame True {
                  }
                }
                n162 = call "Speed Logging-Notifier.vi"("ignore previous (F)"=w176, "error in"=w178, "Timeout waiting in ms (-1)"=w172, "Notifier Function"=Notifier_Function."Wait on notification") -> ("Notification data received"=w175:T20, "Timed out waiting"=w180:bool)  [unwired: 5 in, 1 out]
                n163 = Unbundle By Name(w175) -> ("Log speed data"=w174:bool)
                n164 = Select(t=Speed_logging_states_enum."Log" ("f"), s=w174, f=Speed_logging_states_enum."Close file" ("States")) -> (s? t:f=w182:T2)
                n165 = Select(t=Speed_logging_states_enum."Log", s=w180, f=w182) -> (s? t:f=w179:T2)
              }
              frame "Close file" {
                w202 = TRUE
                n166 = Flush Queue(queue=w199) -> ()  [unwired: 1 in, 3 out]
                n167 = flat-sequence {
                  tunnel: w204 -> [w209]
                  tunnel: w203 -> [w208]
                  tunnel: w202 -> [_]
                  frame #0 {
                    n168 = Close File(refnum=w209, error in=w208) -> (error out=w207:errorcluster)  [unwired: 1 out]
                    n169 = call <vilib>:"Simple Error Handler.vi"("error in (no error)"=w207) -> ("error out"=w206:errorcluster)  [unwired: 4 in, 4 out]
                    n170 = call <vilib>:"Clear Errors.vi"("error in (no error)"=w206) -> ()  [unwired: 5 in, 2 out]
                  }
                }
                "Closed" <- w202
              }
            }
            n171 = Tick Count (ms)() -> (millisecond timer value=w94:u32)
            n172 = feedback #6() -> (w95:u32)  [unwired: 1 in]
            n173 = feedback-in #6(w94) -> ()
            n174 = Subtract(x=w94, y=w95) -> (x-y=→"Logging interval":u32)
            n175 = global read "General Globals.vi" "Stop application"() -> (w90:bool)
            n176 = local read "Stop Button"() -> (w89:bool)
            n177 = Or(x=w90, y=w89) -> (x .or. y?=w88:bool)
            n178 = Select(t=Speed_logging_states_enum."Idle" ("States"), s=w99, f=w97) -> (s? t:f=w98:T2)
            "State" <- w105
            "File path & name" <- w100
          }
          n179 = UDP Close(connection ID=w56, 8:w55) -> (error out=w60:errorcluster)  [unwired: 1 out]
          n180 = flat-sequence {
            tunnel: w68 -> [_]
            tunnel: w67 -> [_]
            tunnel: w65 -> [w211]
            tunnel: w40 -> [_]
            frame #0 {
              n181 = Release Queue(queue=w211) -> ()  [unwired: 2 in, 3 out]
              n182 = local write "Stop Button"(FALSE ("Stop Button")) -> ()
              n183 = call "Speed Graph Window-Notifier.vi"("Notifier Function"=Notifier_Function."Release notifier") -> ()  [unwired: 8 in, 3 out]
              n184 = call "Speed Logging-Notifier.vi"("Notifier Function"=Notifier_Function."Release notifier") -> ()  [unwired: 8 in, 3 out]
            }
          }
          n185 = call <vilib>:"Clear Errors.vi"("error in (no error)"=w60) -> ("error out"=→"Error out (no error)":errorcluster)  [unwired: 5 in, 1 out]
        }
        frame True {
          # "IP address setting is blank"
          n186 = Set Menu Item Info(7:w366, 9:FALSE ("enabled"), 11:w368) -> ()  [unwired: 2 in, 4 out]
          n187 = call "Message Window.vi"("Message string"="To connect to an encoder you must first specify its IP address through the System Configuration window.\n \nThe encoder functionality has been disabled. Update the Encoder setup in the System Configuration window and restart the software.\n") -> ()  [unwired: 10 in, 1 out]
        }
      }
    }
  }
